vi "MPM_Get_Each_Module_Loggdata.vi"(8 "error in (no error)":errorcluster, 10 "moduleNumber":i32, 11 ".NET Reference in":refnum<k24>) -> (0 "error out":errorcluster, 2 "data out":sgl[][](array[numeric]), 3 "Reference out":refnum<k24>)   [LabVIEW 2017]
uses:
  C:/Users/Ssantec_Test/Documents/Instrument_DLL_Sample_Labview_20220902_Ver1.2.2/DLL/x86/InstrumentDLL.dll
  DLL/x86/InstrumentDLL.dll
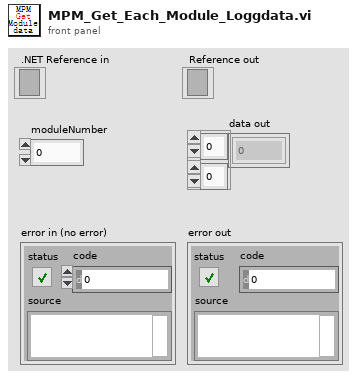
[diagram p1: front panel]
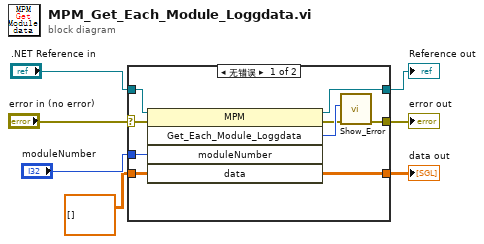
[diagram p0: block diagram]
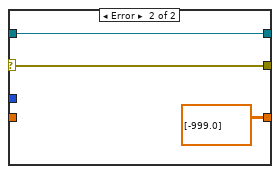
[diagram p2: hidden frame]
diagram:
  n1 = case shown="无错误" "error in (no error)" {
    selector: "error in (no error)" -> [w12 w18]
    tunnel: [w16 sgl[][] [[-999.0]] ("data")] -> w1
    tunnel: "moduleNumber" -> [w15 _]
    tunnel: ".NET Reference in" -> [w14 w19]
    tunnel: [w13 w19] -> w5
    tunnel: [w9 w18] -> w3
    tunnel: sgl[][] [] ("data") -> [w8 _]
    frame No Error {
      n2 = invoke class="MPM" method="Get_Each_Module_Loggdata"(reference=w14, error in=w12, "moduleNumber"=w15, "data"=w8) -> (reference out=w13:refnum<k24>, error out=w10:errorcluster, "Get_Each_Module_Loggdata"=w11:i32, "data"=w16:sgl[][])  [unwired: 1 in, 1 out]
      n3 = call "Show_Error.vi"("error in (no error)"=w10, "Error"=w11) -> ("error out"=w9:errorcluster)  [unwired: 9 in]
    }
    frame Error {
    }
  }
  "Reference out" <- w5
  "error out" <- w3
  "data out" <- w1
